vi "New INI Key for Boolean.vi"(9 "Use ATL":bool=TRUE, 10 "INI key (in)":string="Scan Rats Directory", 11 "INI section (in)":string="File Paths") -> (2 "output cluster":T1={"INI Section"="", "INI Key"="", "Use ATL"=TRUE})   [LabVIEW 2010]
uses:
  <vilib>/Utility/sysdir.llb/System Directory Type.ctl
  <vilib>/Utility/config.llb/Read Key (Boolean).vi
  <vilib>/Utility/config.llb/NI_LVConfig.lvlib
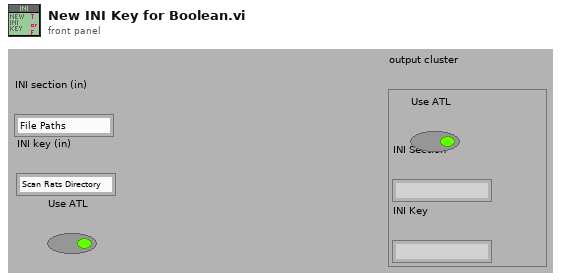
[diagram p1: front panel]
types:
  T1 = cluster{"INI Section":string, "INI Key":string, "Use ATL":bool}
  T2 = cluster{"INI Section":string, "INI Key":string, "Boolean":bool}
  T3 = typedef "System Directory Type.ctl" = i32
  T4 = typedef "NI_LVConfig.lvlib/Config Data RefNum.ctl" = refnum<k1>
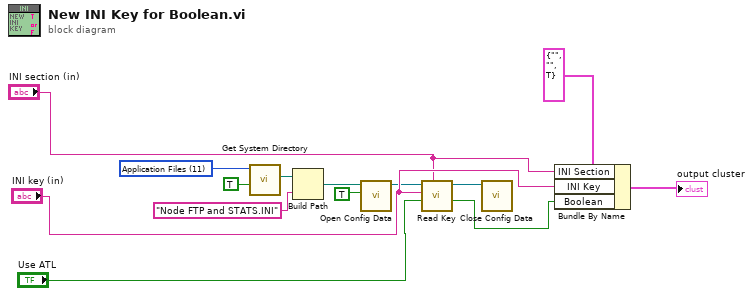
[diagram p0: block diagram]
diagram:
  w6 = T3 11 items=["User Home"=0, "User Desktop"=1, "User Documents"=2, "User Application Data"=3, "User Preferences"=4, "User Temporary"=5, "Public Documents"=6, "Public Application Data"=7, "Public Preferences"=8, "Public Cache"=13, "System Core Libraries"=9, "System Installed Libraries"=10, "Application Files"=11, "Boot Volume Root"=12] ("system directory type")
  n1 = call <vilib>:"Get System Directory.vi"("create directory if not found? (F)"=TRUE, "system directory type"=w6) -> ("system directory"=w7:path)  [unwired: 9 in]
  n2 = Build Path(base path=w7, name or relative path="Node FTP and STATS.INI") -> (appended path=w9:path)
  n3 = call <vilib>:"Open Config Data.vi"("create file if necessary (T)"=TRUE, "configuration file path"=w9) -> ("refnum"=w10:T4)  [unwired: 7 in, 2 out]
  n4 = call-poly <vilib>:"Read Key.vi"("section"="INI section (in)", "default value"="Use ATL", "key"="INI key (in)", "refnum"=w10) -> ("value"=w1:bool, "refnum out"=w11:T4)  [unwired: 4 in, 2 out]
  n5 = call <vilib>:"Close Config Data.vi"("refnum"=w11) -> ()  [unwired: 9 in, 2 out]
  n6 = Bundle By Name(cluster=T2 {"INI Section"="", "INI Key"="", "Boolean"=TRUE} ("output cluster 2"), "INI Section"="INI section (in)", "INI Key"="INI key (in)", "Boolean"=w1) -> (→"output cluster":T2)
